vi "PM-P-calculate_heartreate.vi"(8 "error in (no error)":errorcluster, 11 "loop data":T1) -> (0 "error out":errorcluster, 3 "loop data out":T1)   [LabVIEW 2020]
uses:
  PM-P-loop_data.ctl
  PM-P-user_events.ctl
  init-close/PM-common-heartrate_data.ctl
  <vilib>/measure/matone.llb/Extract Single Tone Information 1 Chan.vi
  <vilib>/measure/NI_MAPro.lvlib
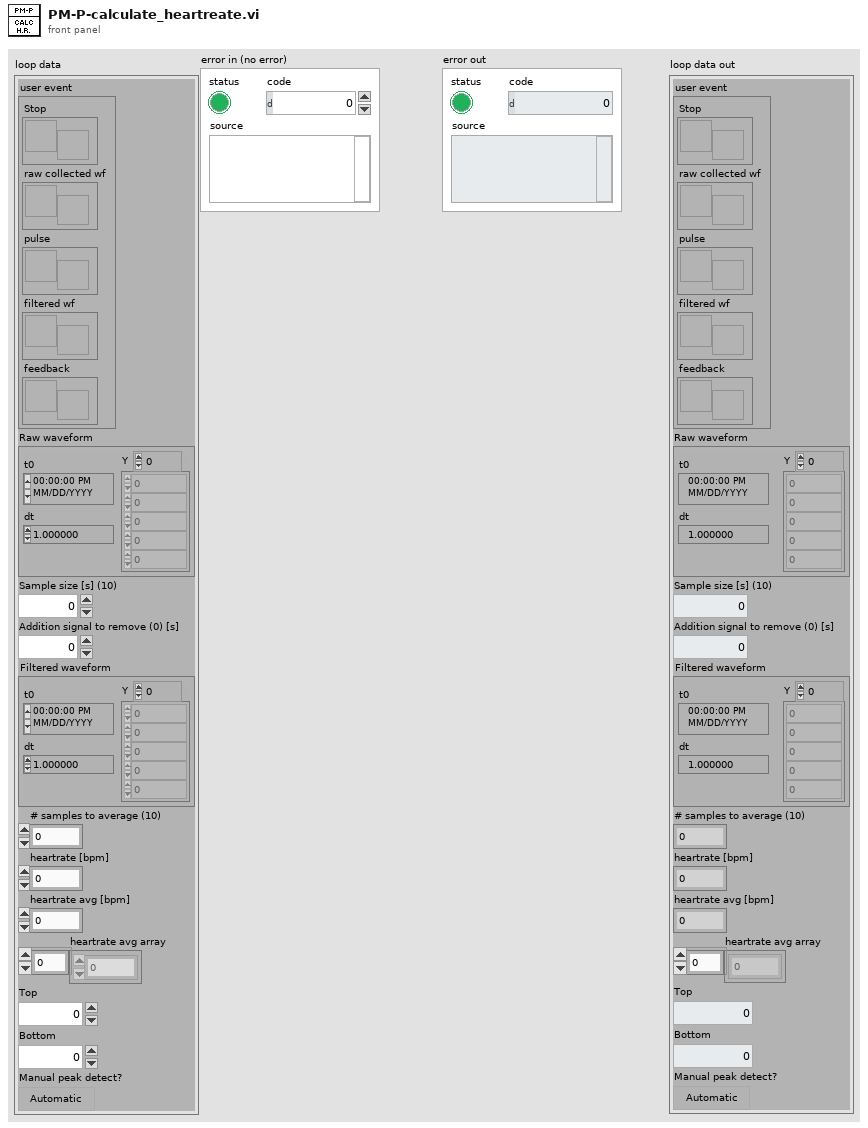
[diagram p1: front panel]
types:
  T1 = typedef "PM-P-loop_data.ctl" = cluster{"user event":T2, "Raw waveform":waveform(dbl), "Sample size [s] (10)":i32, "Addition signal to remove (0) [s]":dbl, "Filtered waveform":waveform(dbl), "# samples to average (10)":i32, "heartrate [bpm]":dbl, "heartrate avg [bpm]":dbl, "heartrate avg array":dbl[], "Top":dbl, "Bottom":dbl, "Manual peak detect?":bool}
  T2 = typedef "PM-P-user_events.ctl" = cluster{"Stop":refnum<user-event>, "raw collected wf":refnum<user-event>, "pulse":refnum<user-event>, "filtered wf":refnum<user-event>, "feedback":refnum<user-event>}
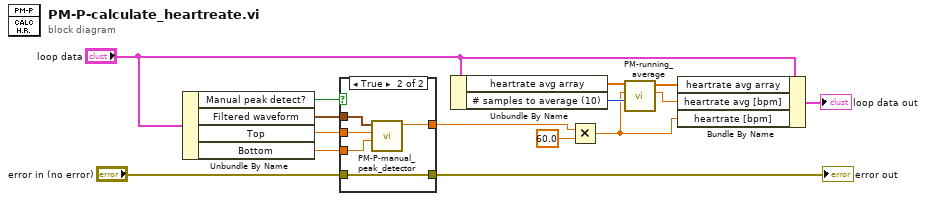
[diagram p0: block diagram]
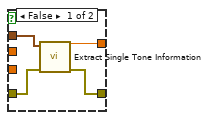
[diagram p2: hidden frame]
diagram:
  n1 = Unbundle By Name("loop data") -> ("Manual peak detect?"=w4:bool, "Filtered waveform"=w3:waveform(dbl), "Top"=w2:dbl, "Bottom"=w1:dbl)
  n2 = case shown="True" w4 {
    tunnel: [w19 w21] -> w14
    tunnel: "error in (no error)" -> [w18 w20]
    tunnel: [w17 w20] -> w8
    tunnel: w3 -> [w16 w24]
    tunnel: w2 -> [_ w23]
    tunnel: w1 -> [_ w22]
    frame False {
      n3 = call-poly <vilib>:"Extract Single Tone Information.vi"("error in (no error)"=w18, "time signal in"=w16) -> ("error out"=w17:errorcluster, "detected frequency"=w19:dbl)  [unwired: 4 in, 4 out]
    }
    frame True {
      n4 = call "PM-P-manual_peak_detector.vi"("Bot"=w22, "Top"=w23, "waveform in"=w24) -> ("Frequency [Hz]"=w21:dbl)  [unwired: 7 in, 1 out]
    }
  }
  "error out" <- w8
  n5 = Unbundle By Name("loop data") -> ("heartrate avg array"=w6:dbl[], "# samples to average (10)"=w12:i32)
  n6 = Multiply(x=w14, y=60.0) -> (x*y=w9:dbl)
  n7 = call "PM-running_average.vi"("Average over (10)"=w12, "new value"=w9, "value array in"=w6) -> ("Average"=w10:dbl, "value array out"=w7:dbl[])  [unwired: 6 in, 1 out]
  n8 = Bundle By Name(cluster="loop data", "heartrate avg array"=w7, "heartrate avg [bpm]"=w10, "heartrate [bpm]"=w9) -> (→"loop data out":T1)
